vi "traceFileIO_readFromFile_index.vi"(0 "reference":refnum<class "OSA.lvclass">, 1 "path":path, 2 "file_trace idx":u32, 3 "dataType":T1, 4 "trace idx":u32, 5 "error in (no error)":errorcluster, 7 "dialog (empty path)":bool) -> (14 "duplicate reference":refnum<class "OSA.lvclass">, 17 "cancelled":bool, 19 "error out":errorcluster)   [LabVIEW 2010, in "OSA.lvclass"]
doc: "Reads trace data from spf2 binary file and store into trace buffer. This routine supports spf2 file with more than one trace."
uses:
  OSA.lvclass
  typeDef/trace_properties_ui.ctl
  typeDef/acq_dataType.ctl
  OSA20X_misc.lvlib
  FTSLib.dll
panel:
  out "trace log 2":string
  out "trace log":string
  in  "property":T2=enum."type"
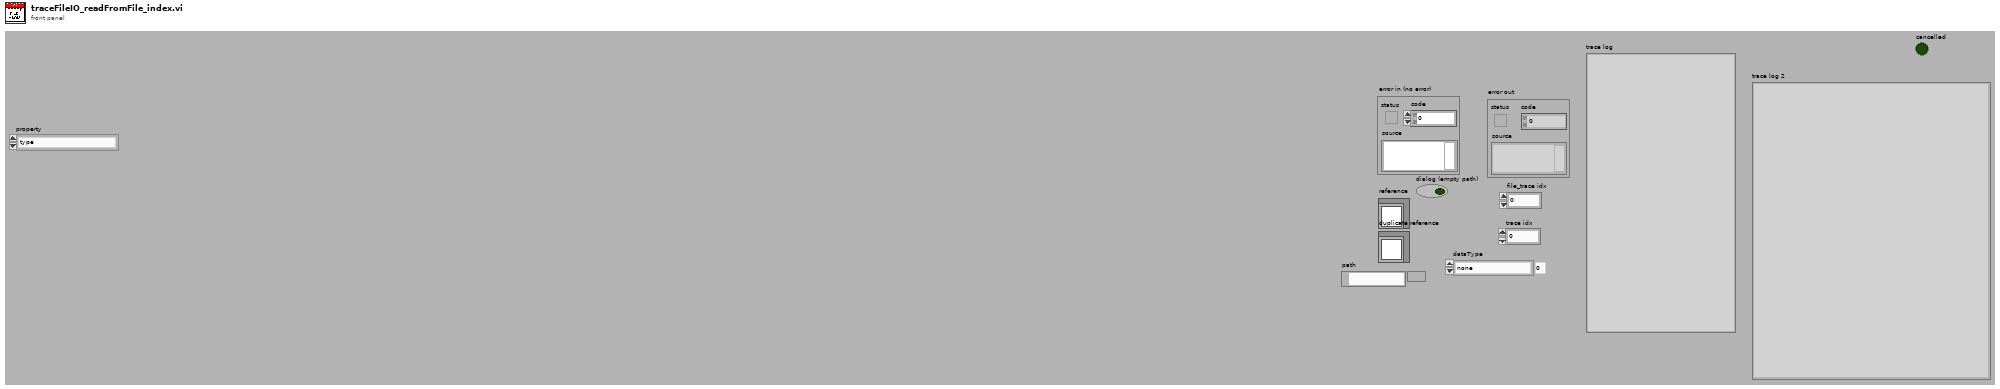
[diagram p1: front panel]
types:
  T1 = typedef "OSA.lvclass/acq_dataType.ctl" = enum16{"none", "interferogram", "spectrum"}
  T2 = typedef "OSA.lvclass/trace_properties_ui.ctl" = enum16{"length", "type", "acquisitionMode", "xValueFormat", "date", "time", "averageNum", "smoothType", "igramSmoothType", "phaseCorrection", "apodisation", "__allocatedLengthI", "__allocatedLengthx", "adcBits", "sensitivityMode", "resolutionMode", "rollingAverage", "samplesPerReference", "air_measureOption", "interferogramProperty", "all_uiProperties"}
  T3 = enum16{"length", "type", "acquisitionMode", "xValueFormat", "date", "time", "averageNum", "smoothType", "igramSmoothType", "phaseCorrection", "apodisation", "__allocatedLengthI", "__allocatedLengthx", "adcBits", "sensitivityMode", "resolutionMode", "rollingAverage", "samplesPerReference", "air_measureOption", "interferogramProperty", "all_uiProperties"}
  T4 = typedef "OSA.lvclass/ObjectAttributes.ctl" = cluster{"Stop":bool, "dataType":T1, "spectrometerIdx":u16, "buffer size interferogram":i32, "interferogram":cluster{"new":bool, "plot_x_ min":sgl, "plot_x_max":sgl, "plot_y_min":sgl, "plot_y_max":sgl, "Graph Intrfrgrm":T5, "timeStamp":u32, "signal (%)":dbl, "traces":cluster{"idx":u32, "broadBand":bool, "monoChromatic":bool, "peakToPeakSignal":dbl, "peakToPeakPos":dbl}[], "traces idx last":i32}, "spectrum":cluster{"new":bool, "plot_x_min":sgl, "plot_x_max":sgl, "plot_unit_x":T6, "plot_unit_y":T7, "plot_y_min":sgl, "plot_y_max":sgl, "Graph Spectrum":T5, "timeStamp":u32, "X_VAL_OPTIONS":enum16{"MIN_MAX", "ARRAY"}, "traces":cluster{"idx":u32}[], "traces idx last":i32}, "Thorlabs_OSA_64.lvclass:queue_action.ctlqueue ref":refnum<queue>, "action":T8, "plot zoom step":dbl, "buffer semaphore":T9, "acq stopped":bool, "dataType active":T1, "temperature (degr C)":sgl, "pressure (hPa)":sgl, "rel humidity (%)":sgl, "settings":cluster{"resolution":u16, "sensitivity":u16, "Average":bool, "average nr":u32, "apodisation":T10, "acq delay (ms)":u32, "airMesure":T11, "wmtr on":bool, "intfgrm_smooth_width":u16, "intfgrm_smooth_nrOfPasses":u16, "intfgrm_smooth":T12, "phaseCorrection":T13, "zeroFill":u8, "spectr_smooth":T12, "spectr_smooth_width":u16, "spectr_smooth_nrOfPasses":u16, "resolution (/cm)":sgl, "REF wavelength, (nm)":dbl, "gain_idx":u16, "gainAuto":bool, "gain_relative":dbl, "PD sensitivity mode":T14, "PD senseMode implemented":bool, "SensorTemperature implemented":bool, "SensorPressure implemented":bool, "SensorHumidity implemented":bool, "attenuationAuto":bool, "attenuationOnOff":bool, "attenuationAvailable":bool, "offsetAvailable":bool, "offset":i32, "offset max":u16}, "peaks position":sgl[], "peaks width":sgl[], "peaks height":sgl[], "peaks max nr":u32, "peaks latest nr":i32, "peaks new":bool, "power":dbl, "power new":bool, "path":string, "wavelength (WNr)":dbl, "wavelength new":bool, "buffer size spectrum":i32, "status":string, "VI reference":refnum<vi>, "funcPointer":u64, "libraryPointer":u64, "singleAcquisition":bool, "coherenceLength (cm)":dbl, "coherenceLength new":bool, "spectrometer model":string, "spectrometer serial nr":string, "peaks thld left":sgl[], "peaks thld right":sgl[], "coherenceLength error (cm)":dbl, "ADC bits":u16, "peaks position centroid":sgl[], "peaks height centroid":sgl[], "OSA series":T15, "channel index spectrum":u16, "spectrometer rangeLow, (/cm)":dbl, "spectrometer rangeHigh, (/cm)":dbl, "channel index interferogram":u16}
  T5 = typedef "OSA.lvclass/graph_intensity.ctl" = refnum<vi>
  T6 = typedef "OSA.lvclass/spectrum_x_unit.ctl" = enum16{"wavenr/cm", "THz", "eV", "nm_air", "nm_vac"}
  T7 = typedef "OSA.lvclass/y_unit.ctl" = enum16{"ADC counts", "dBm pwr absolute", "dBm pwr density", "mW pwr absolute", "mW pwr density"}
  T8 = typedef "OSA.lvclass/queue_action.ctl" = enum16{"none", "stop", "GUI_plotInterferogram", "GUI_plotSpectrum", "GUI_plotInterferogramRescale", "GUI_plotSpectrumRescale", "GUI_plotInterferogramReset", "GUI_plotSpectrumReset", "GUI_plotInterferogramAutoScaleY", "GUI_plotSpectrumAutoScaleY", "GUI_plotInterferogramZoomOut", "GUI_plotSpectrumZoomOut", "GUI_plotInterferogramPane", "GUI_plotSpectrumPane", "GUI_plotInterferogramZoomMouse", "GUI_plotSpectrumZoomMouse", "GUI_spectrumChannelType", "GUI_channel", "ENVIRONMENT temperature", "ENVIRONMENT pressure", "MODE_resolution set", "MODE_resolution get", "MODE_sensitivity set", "MODE_sensitivity get", "MODE_PDTemperature set", "MODE_PDTemperature get", "REBOOT/RESET firmware", "ACQASYNC_acquireSingleSpectrum", "ACQASYNC_continuous start", "ACQASYNC_continuous stop\n", "ACQASYNC_get last interferogram", "ACQASYNC_get last spectrum", "ACQASYNC_get last waveNr", "ACQOPT_interferogram smoothing set", "ACQOPT_interferogram smoothing get", "ACQOPT_spectrum smoothing set", "ACQOPT_spectrum smoothing get", "ACQOPT_apodisation type set", "ACQOPT_apodisation type get", "ACQOPT_phase correction type set", "ACQOPT_phase correction type get", "ACQOPT_acqIntervall_set", "ACQOPT_acqIntervall_get", "ACQOPT_average spectrum set", "ACQOPT_average spectrum get", "ACQOPT_rolling average set", "ACQOPT_rolling average get", "ACQOPT_zero fill factor set", "ACQOPT_zero fill factor get", "ACQOPT_cycle counting set", "ACQOPT_cycle counting get", "ACQOPT_air measure option set", "ACQOPT_air measure option get", "ACQOPT_gainLevel auto get", "ACQOPT_gainLevel auto set", "ACQOPT_gainLevel get", "ACQOPT_gainLevel set", "ACQOPT_getAll", "INSTRUMENT_PROPERTY_range_WaveNr_min", "INSTRUMENT_PROPERTY_range_WaveNr_max", "INSTRUMENT_PROPERTY_reference_wavelength_cm^-1", "INSTRUMENT_PROPERTY_samplesPerRefPeriod", "INSTRUMENT_PROPERTY_resolution_waveNrPercm", "INSTRUMENT_PROPERTY_availableGainLevels", "INSTRUMENT_PROPERTY_status", "CONVERT", "ANALYSE_POWER", "ANALYSE_PEAKS", "ANALYSE_WAVELENGTH", "ANALYSE_SPECTRUM", "ANALYSE_INTERFEROGRAM", "ANALYSE_COHERENCE_LENGTH", "MATH", "MATH_power", "MATH_peaks", "FILE", "miscellaneous"}
  T9 = typedef "Semaphore RefNum" = refnum<k1>
  T10 = typedef "OSA.lvclass/apodisation.ctl" = enum16{"NONE", "NORTON_BEER_WEAK", "NORTON_BEER_MEDIUM", "NORTON_BEER_STRONG", "TRIANGULAR", "COSINE", "HANN", "HAMMING", "BLACKMANHARRIS3", "BLACKMANHARRIS4", "GAUSSIAN"}
  T11 = typedef "OSA.lvclass/airMeasure.ctl" = enum16{"TEMPERATURE", "PRESSURE"}
  T12 = typedef "OSA20X_misc.lvlib/interferogram_smoothing.ctl" = enum16{"NONE", "BINOMIAL", "SAVITSKY_GOLAY", "FOURIER", "MOVING_AVERAGE", "GAUSSIAN"}
  T13 = typedef "OSA.lvclass/phaseCorrection.ctl" = enum16{"NONE", "MERTZ", "FORMAN", "MERTZ_FILE", "FORMAN_FILE", "FUTURE COMP."}
  T14 = typedef "OSA20X_misc.lvlib/PDTemperatureMode.ctl" = enum16{"cool: better sensitivity/noise floor", "warm: extended wl range"}
  T15 = typedef "OSA.lvclass/OSA_series.ctl" = enum16{"OSA200", "OSA300", "UNKNOWN"}
  T16 = cluster{"idx":u32, "broadBand":bool, "monoChromatic":bool, "peakToPeakSignal":dbl, "peakToPeakPos":dbl}[]
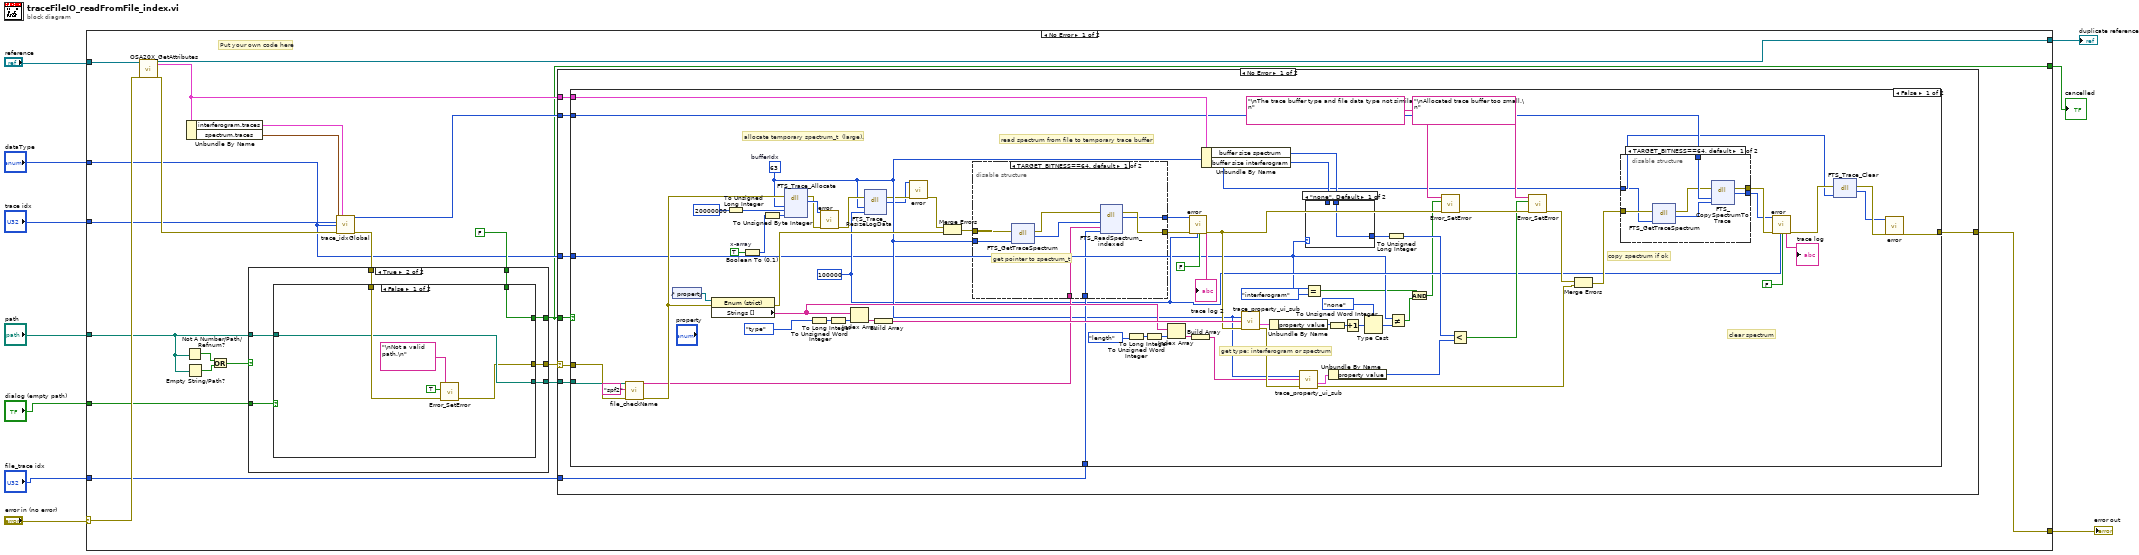
[diagram p0: block diagram]
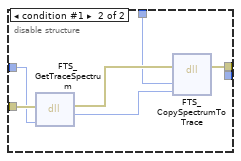
[diagram p2: hidden frame]
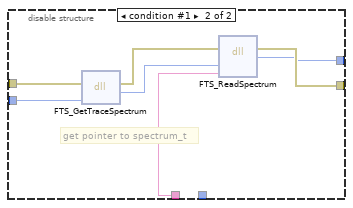
[diagram p4: hidden frame]
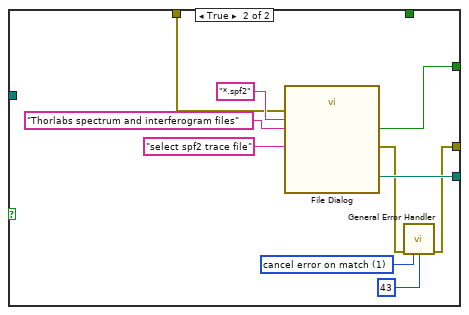
[diagram p8: hidden frame]
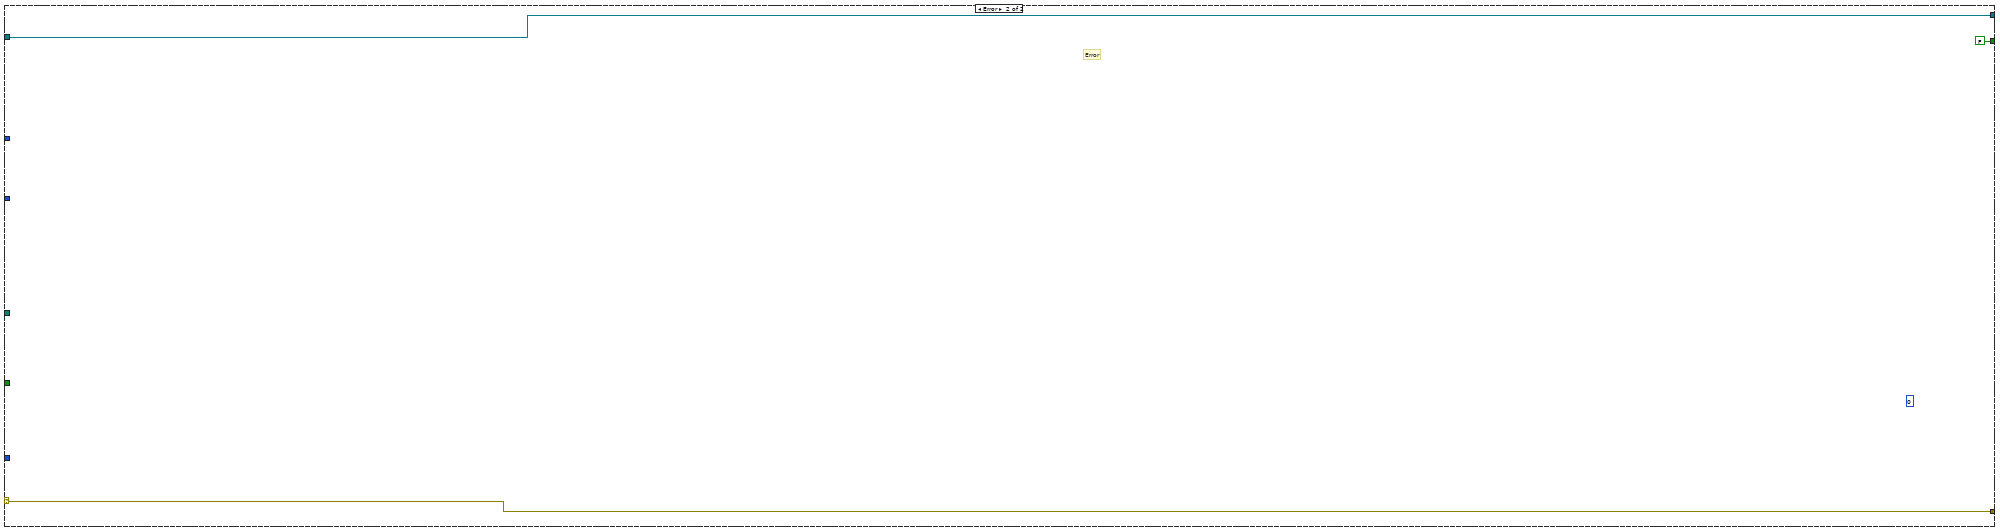
[diagram p9: hidden frame]
diagram:
  n1 = case shown="No Error" "error in (no error)" {
    selector: "error in (no error)" -> [w31 w174]
    tunnel: [w21 w174] -> w9
    tunnel: "reference" -> [w32 w173]
    tunnel: [w22 w173] -> w7
    tunnel: "trace idx" -> [w15 _]
    tunnel: "path" -> [w16 _]
    tunnel: "dataType" -> [w14 _]
    tunnel: "dialog (empty path)" -> [w13 _]
    tunnel: "file_trace idx" -> [w12 _]
    tunnel: [w11 FALSE ("cancelled")] -> w1
    frame No Error {
      # "Put your own code here"
      n2 = call "OSA20X_GetAttributes.vi"("reference in"=w32, "error in (no error)"=w31) -> ("reference out"=w22:refnum<class "OSA.lvclass">, "Data"=w18:T4, "error out"=w17:errorcluster)  [unwired: 14 in, 1 out]
      n3 = Not A Number/Path/Refnum?(number/path/refnum=w16) -> (NaN/Path/Refnum?=w29:bool)
      n4 = Empty String/Path?(string/path=w16) -> (empty?=w30:bool)
      n5 = Unbundle By Name(w18) -> ("interferogram.traces"=w20:T16, "spectrum.traces"=w19:cluster{"idx":u32}[])
      n6 = Or(x=w29, y=w30) -> (x .or. y?=w28:bool)
      n7 = call "trace_idxGlobal.vi"("traces_spectrum"=w19, "traces_interferogram"=w20, "trace idx"=w15, "dataType"=w14, "error in (no error)"=w17) -> ("global trace idx"=w27:u32, "error out"=w26:errorcluster)  [unwired: 9 in]
      n8 = case shown="True" w28 {
        tunnel: w16 -> [w147 w151]
        tunnel: w13 -> [_ w155]
        tunnel: w26 -> [w148 w154]
        tunnel: [w146 w152] -> w11
        tunnel: [w147 w153] -> w24
        tunnel: [w148 w150] -> w25
        tunnel: FALSE ("cancelled") -> [w146 w149]
        frame False {
        }
        frame True {
          n9 = case shown="False" w155 {
            tunnel: w154 -> [w161 w168]
            tunnel: [w158 w167] -> w153
            tunnel: [w156 w166] -> w152
            tunnel: w151 -> [w158 _]
            tunnel: [w157 w162] -> w150
            tunnel: w149 -> [w156 _]
            frame False {
              n10 = call "Error_SetError.vi"("error in"=w161, "status (true)"=TRUE, "source(\"\")"="\nNot a valid path.\n" ("source(\"\")")) -> ("error out"=w157:errorcluster)  [unwired: 4 in]
            }
            frame True {
              w165 = 1 items=["no exception", "cancel error on match", "set error on match"] ("[exception action] (none:0)")
              n11 = call "File Dialog"("prompt"="select spf2 trace file", "error in"=w168, "pattern (all files)"="*.spf2", "pattern label"="Thorlabs spectrum and interferogram files") -> ("selected path"=w167:path, "cancelled"=w166:bool, "error out"=w163:errorcluster)  [unwired: 8 in, 1 out]
              n12 = call <vilib>:"General Error Handler.vi"("error in (no error)"=w163, "[exception action] (none:0)"=w165, "[exception code]"=43) -> ("error out"=w162:errorcluster)  [unwired: 8 in, 4 out]
            }
          }
        }
      }
      n13 = case shown="No Error" w25 {
        selector: w25 -> [w38 w145]
        tunnel: w27 -> [w40 _]
        tunnel: [w39 w145] -> w21
        tunnel: w11 -> [w36 _]
        tunnel: w24 -> [w37 _]
        tunnel: w14 -> [w35 _]
        tunnel: w18 -> [w34 _]
        tunnel: w12 -> [w33 _]
        frame No Error {
          n14 = case shown="False" w36 {
            tunnel: w40 -> [w71 _]
            tunnel: [w57 w144] -> w39
            tunnel: w38 -> [w65 w144]
            tunnel: w37 -> [w64 _]
            tunnel: w35 -> [w45 _]
            tunnel: w34 -> [w81 _]
            tunnel: w33 -> [w60 _]
            frame False {
              w46 = u32 100000 ("size")
              w111 = TRUE  # x-array
              w52 = u32 63  # bufferIdx
              # "clear spectrum"
              # "copy spectrum if ok"
              # "get type: interferogram or spectrum"
              # "read spectrum from file to temporary trace buffer"
              # "allocate temporary spectrum_t  (large)."
              n15 = call "file_checkName.vi"("path"=w64, "filename extension"="spf2", "error in (no error)"=w65) -> ("path string out"=w61:string, "error out"=w62:errorcluster)  [unwired: 13 in, 2 out]
              n16 = control-ref of="property"() -> (w106:refnum<vi>)
              n17 = property class="Enum (strict)"(reference=w106, error in=w62) -> (error out=w100:errorcluster, "Strings []"=w85:string[])  [unwired: 1 out]
              n18 = To Unsigned Long Integer(number=u32 20000000) -> (unsigned 32bit integer=w112:u32)
              n19 = Boolean To (0,1)(Boolean=w111) -> (0, 1=w110:i16)
              n20 = To Unsigned Byte Integer(number=w110) -> (unsigned 8bit integer=w109:u8)
              n21 = dll-call lib="FTSLib.dll" fn="FTS_Trace_Allocate"(error in=w62, "bufferIdx"=w52, "spectrumLength"=w112, "addX"=w109) -> (error out=w107:errorcluster, "returnValue"=w108:i32)  [unwired: 5 in, 1 out]
              n22 = To Unsigned Word Integer(number=T3."type" ("Value")) -> (unsigned 16bit integer=w105:u16)
              n23 = call "error.vi"("result code"=w108, "error in (no error)"=w107) -> ("error out"=w53:errorcluster)  [unwired: 15 in, 2 out]
              n24 = To Long Integer(number=w105) -> (32bit integer=w104:i32)
              n25 = Index Array(array=w85, index=w104) -> (element=w103:string)
              n26 = dll-call lib="FTSLib.dll" fn="FTS_Trace_ResizeLogData"(error in=w53, "bufferIdx"=w52, "size"=w46) -> (error out=w51:errorcluster, "returnValue"=w50:i32)  [unwired: 4 in, 1 out]
              n27 = Build Array(w103) -> (w102:string[])
              n28 = call "error.vi"("result code"=w50, "error in (no error)"=w51) -> ("error out"=w49:errorcluster)  [unwired: 15 in, 2 out]
              n29 = Merge Errors(w49, w100) -> (w99:errorcluster)
              n30 = disable-structure shown="TARGET_BITNESS==64, default" {
                disable-tunnel: w52 -> [w131 w140]
                disable-tunnel: w61 -> [w136 w139]
                disable-tunnel: w99 -> [w134 w141]
                disable-tunnel: [w133 w138] -> w113
                disable-tunnel: [w132 w137] -> w101
                disable-tunnel: w60 -> [w129 _]
                frame condition #0 (active) {
                  # "get pointer to spectrum_t"
                  n31 = dll-call lib="FTSLib.dll" fn="FTS_GetTraceSpectrum"(error in=w134, "traceIdx"=w131) -> (error out=w135:errorcluster, "spectrum_t_pointer"=w130:u64)  [unwired: 3 in, 1 out]
                  n32 = dll-call lib="FTSLib.dll" fn="FTS_ReadSpectrum_indexed"(error in=w135, "spectrum_t_pointer"=w130, "fileNameAndPath"=w136, "trace_idx"=w129) -> (error out=w133:errorcluster, "returnValue"=w132:i32)  [unwired: 5 in, 1 out]
                }
                frame condition #1 {
                  # "get pointer to spectrum_t"
                  n33 = dll-call lib="FTSLib.dll" fn="FTS_GetTraceSpectrum"(error in=w141, "traceIdx"=w140) -> (error out=w142:errorcluster, "spectrum_t_pointer"=w143:u32)  [unwired: 3 in, 1 out]
                  n34 = dll-call lib="FTSLib.dll" fn="FTS_ReadSpectrum"(error in=w142, "spectrum_t_pointer"=w143, "fileNameAndPath"=w139) -> (error out=w138:errorcluster, "parameter"=w137:i32)  [unwired: 4 in, 1 out]
                }
              }
              n35 = To Unsigned Word Integer(number=T3."length" ("Value")) -> (unsigned 16bit integer=w89:u16)
              n36 = To Long Integer(number=w89) -> (32bit integer=w88:i32)
              n37 = Index Array(array=w85, index=w88) -> (element=w87:string)
              n38 = call "error.vi"("result code"=w101, "error in (no error)"=w113, "size trace log"=w46, "call trace log"=FALSE) -> ("trace log"=→"trace log 2":string, "error out"=w93:errorcluster)  [unwired: 13 in, 1 out]
              n39 = Build Array(w87) -> (w84:string[])
              n40 = Unbundle By Name(w81) -> ("buffer size spectrum"=w75:i32, "buffer size interferogram"=w76:i32)
              n41 = call "trace_property_ui_sub.vi"("trace idx global"=w52, "properties ui"=w102, "error in (no error)"=w93) -> ("property"=w98:cluster{"property":string, "property value":u32}, "error out"=w91:errorcluster)  [unwired: 10 in, 1 out]
              n42 = Unbundle By Name(w98) -> ("property value"=w97:u32)
              n43 = call "trace_property_ui_sub.vi"("trace idx global"=w52, "properties ui"=w84, "error in (no error)"=w91) -> ("property"=w83:cluster{"property":string, "property value":u32}, "error out"=w67:errorcluster)  [unwired: 10 in, 1 out]
              n44 = Equal?(x=w45, y=acq_dataType."interferogram") -> (x = y?=w43:bool)
              n45 = case shown="\"none\", Default" w45 {
                tunnel: w76 -> [_ w128]
                tunnel: w75 -> [w127 _]
                tunnel: [w127 w128] -> w74
                frame "none", Default {
                }
                frame "interferogram" {
                }
              }
              n46 = To Unsigned Word Integer(number=w97) -> (unsigned 16bit integer=w95:u16)
              n47 = Unbundle By Name(w83) -> ("property value"=w80:u32)
              n48 = Increment(x=w95) -> (x+1=w94:u16)
              n49 = Type Cast(type=acq_dataType."none" ("dataType"), x=w94) -> (*(type *) &x=w82:T1)
              n50 = To Unsigned Long Integer(number=w74) -> (unsigned 32bit integer=w73:u32)
              n51 = Not Equal?(x=w45, y=w82) -> (x != y?=w42:bool)
              n52 = And(x=w43, y=w42) -> (x .and. y?=w41:bool)
              n53 = call "Error_SetError.vi"("error in"=w93, "status (true)"=w41, "source(\"\")"="\nThe trace buffer type and file data type not similar.\n" ("source(\"\")")) -> ("error out"=w79:errorcluster)  [unwired: 4 in]
              n54 = Less?(x=w73, y=w80) -> (x < y?=w72:bool)
              n55 = call "Error_SetError.vi"("error in"=w79, "status (true)"=w72, "source(\"\")"="\nAllocated trace buffer too small.\n" ("source(\"\")")) -> ("error out"=w68:errorcluster)  [unwired: 4 in]
              n56 = Merge Errors(w68, w67) -> (w66:errorcluster)
              n57 = disable-structure shown="TARGET_BITNESS==64, default" {
                disable-tunnel: w66 -> [w120 w126]
                disable-tunnel: [w118 w124] -> w70
                disable-tunnel: [w114 _] -> w69
                disable-tunnel: w52 -> [w119 w125]
                disable-tunnel: w71 -> [w117 w122]
                frame condition #0 (active) {
                  n58 = dll-call lib="FTSLib.dll" fn="FTS_GetTraceSpectrum"(error in=w120, "traceIdx"=w119) -> (error out=w115:errorcluster, "spectrum_t_pointer"=w116:u64)  [unwired: 3 in, 1 out]
                  n59 = dll-call lib="FTSLib.dll" fn="FTS_CopySpectrumToTrace"(error in=w115, "traceBufferIdx_to"=w117, "spectrum_t_pointer_from"=w116) -> (error out=w118:errorcluster, "returnValue"=w114:i32)  [unwired: 4 in, 1 out]
                }
                frame condition #1 {
                  n60 = dll-call lib="FTSLib.dll" fn="FTS_GetTraceSpectrum"(error in=w126, "traceIdx"=w125) -> (error out=w123:errorcluster, "spectrum_t_pointer"=w121:u32)  [unwired: 3 in, 1 out]
                  n61 = dll-call lib="FTSLib.dll" fn="FTS_CopySpectrumToTrace"(error in=w123, "traceBufferIdx_to"=w122, "spectrum_t_pointer_from"=w121) -> (error out=w124:errorcluster)  [unwired: 5 in, 1 out]
                }
              }
              n62 = call "error.vi"("result code"=w69, "error in (no error)"=w70, "size trace log"=w46, "call trace log"=FALSE) -> ("trace log"=→"trace log":string, "error out"=w59:errorcluster)  [unwired: 13 in, 1 out]
              n63 = dll-call lib="FTSLib.dll" fn="FTS_Trace_Clear"(error in=w59, "bufferIdx"=w52) -> (error out=w58:errorcluster, "returnValue"=w56:i32)  [unwired: 3 in, 1 out]
              n64 = call "error.vi"("result code"=w56, "error in (no error)"=w58) -> ("error out"=w57:errorcluster)  [unwired: 15 in, 2 out]
            }
            frame True {
            }
          }
        }
        frame Error {
        }
      }
    }
    frame Error {
      (unwired) u32 0 ("property value")
      # "Error"
    }
  }
  "error out" <- w9
  "duplicate reference" <- w7
  "cancelled" <- w1
